vi "종합1.vi"() -> ()   [LabVIEW 2020]
panel:
  out "흥분도":dbl format="%.2g"
  out "행복도":dbl format="%.2g"
  out "XY Graph":cluster{"Y":dbl[], "Y":dbl[]}[](graph) caption="XY 그래프"
  in  "숫자형 5":dbl
  in  "숫자형 4":dbl
  in  "숫자형 3":dbl
  in  "숫자형 2":dbl
  in  "숫자형":dbl
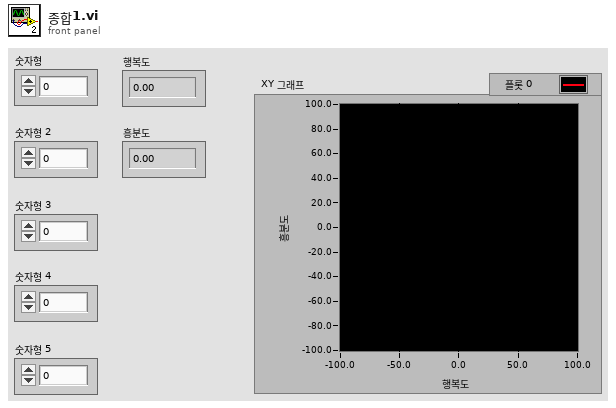
[diagram p1: front panel]
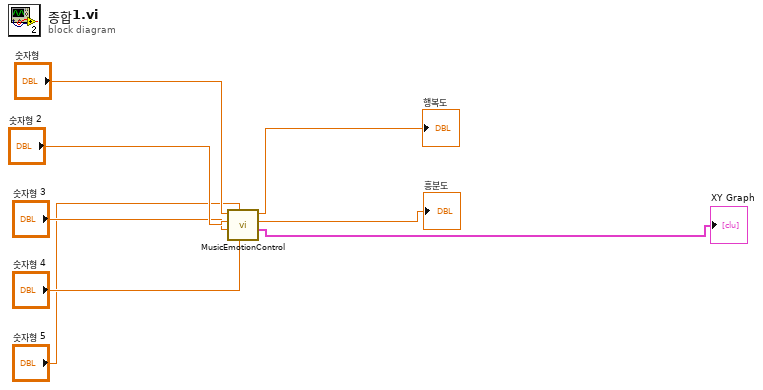
[diagram p0: block diagram]
diagram:
  n1 = call "MusicEmotionControl.vi"("Roll off"="숫자형 4", "Centroid"="숫자형 5", "Zero Crossing"="숫자형 3", "RMS"="숫자형 2", "BPM"="숫자형") -> ("XY Graph"=→"XY Graph":cluster{"Y":dbl[], "Y":dbl[]}[], "흥분도"=→"흥분도":dbl, "행복도"=→"행복도":dbl)  [unwired: 4 in]
